vi "GetType.vi"(8 "error in (no error)":errorcluster, 11 "Create Arbitrary Waveform [ARB] Msg":refnum<class "Create Arbitrary Waveform [ARB] Msg.lvclass">) -> (0 "error out":errorcluster, 2 "Data Sample":variant, 3 "Create Arbitrary Waveform [ARB] Msg":refnum<class "Create Arbitrary Waveform [ARB] Msg.lvclass">)   [LabVIEW 2015, in "CS++Fgen.lvlib" / "Create Arbitrary Waveform [ARB] Msg.lvclass"]
doc: "This VI delivers a sample of the data type format the message expects."
uses:
  Create Arbitrary Waveform [ARB] Msg.lvclass
  Create Arbitrary Waveform [ARB] Msg.lvclass/Create Arbitrary Waveform [ARB] Msg.ctl
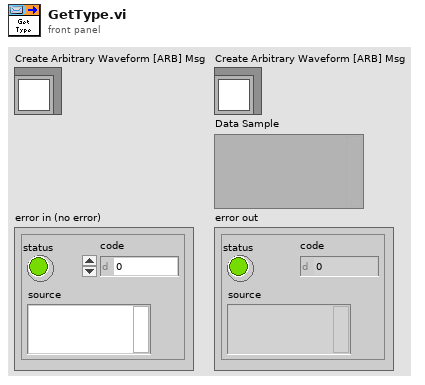
[diagram p1: front panel]
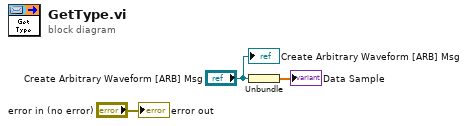
[diagram p0: block diagram]
diagram:
  n1 = Unbundle("Create Arbitrary Waveform [ARB] Msg") -> (→"Data Sample":dbl[])
  "error out" <- "error in (no error)"
  "Create Arbitrary Waveform [ARB] Msg" <- "Create Arbitrary Waveform [ARB] Msg"
